vi "CurrentOutput_nano.vi"(7 "y scaled":dbl, 9 "array":dbl[][](array[numeric]), 10 "Z Input":dbl, 11 "X Input":dbl) -> (0 "Origin":dbl, 1 "FW":dbl, 2 "FH":dbl, 3 "Current Out (pA)":dbl, 4 "Zread":dbl)   [LabVIEW 2017]
uses:
  <vilib>/ptbypt/NI_PtbyPt.lvlib
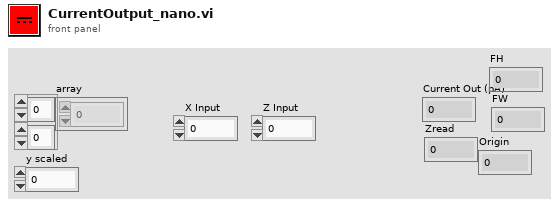
[diagram p1: front panel]
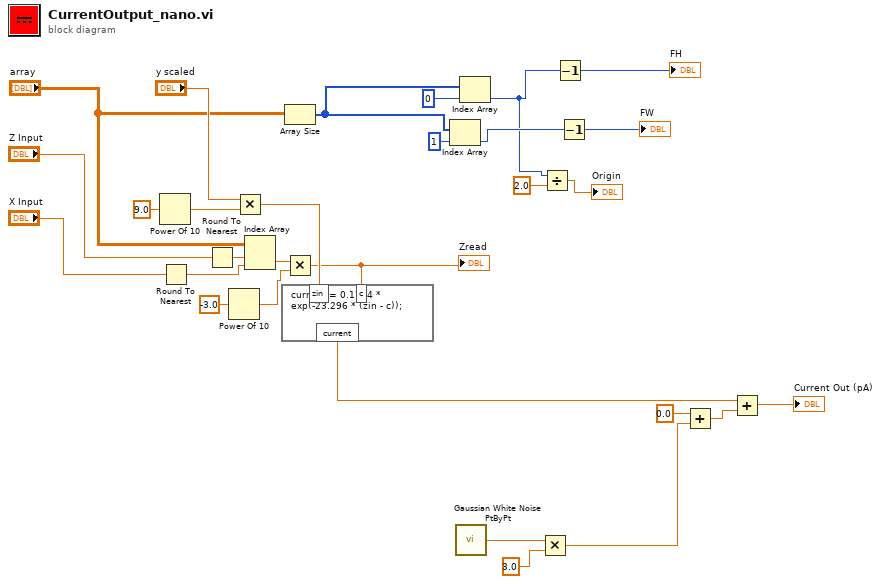
[diagram p0: block diagram]
diagram:
  n1 = Power Of 10(x=9.0) -> (10^x=w28:dbl)
  n2 = Round To Nearest(number="X Input") -> (nearest integer value=w22:dbl)
  n3 = Round To Nearest(number="Z Input") -> (nearest integer value=w29:dbl)
  n4 = Power Of 10(x=-3.0) -> (10^x=w24:dbl)
  n5 = Multiply(x="y scaled", y=w28) -> (x*y=w26:dbl)
  n6 = Index Array(array="array", index (row)=w29, index (col)=w22) -> (element=w19:dbl)
  n7 = Array Size(array="array") -> (size(s)=w14:i32[])
  n8 = Multiply(x=w19, y=w24) -> (x*y=w23:dbl)
  "Zread" <- w23
  n9 = formula code="current = 0.1714 * exp(-23.296 * (zin - c));"("zin"=w26, "c"=w23) -> ("current"=w1:dbl)
  n10 = Index Array(array=w14, index=1) -> (element=w13:i32)
  n11 = call <vilib>:"Gaussian White Noise PtByPt.vi"() -> ("Gaussian white noise"=w7:dbl)  [unwired: 3 in]
  n12 = Index Array(array=w14, index=0) -> (element=w11:i32)
  n13 = Multiply(x=w7, y=3.0) -> (x*y=w4:dbl)
  n14 = Divide(x=w11, y=2.0) -> (x/y=→"Origin":dbl)
  n15 = Decrement(x=w11) -> (x-1=→"FH":i32)
  n16 = Decrement(x=w13) -> (x-1=→"FW":i32)
  n17 = Add(x=0.0, y=w4) -> (x+y=w5:dbl)
  n18 = Add(x=w1, y=w5) -> (x+y=→"Current Out (pA)":dbl)
